vi "UV-VIS GetNumberHSSpeedsSD.vi"(4 "error in (no error)":errorcluster, 5 "type":T1, 6 "channel":i32, 7 "Control in":refnum<class "CCD_camera.lvclass">) -> (0 "error out":errorcluster, 1 "DLL error code":u32, 2 "number":i32, 3 "Control out":refnum<class "CCD_camera.lvclass">)   [LabVIEW 2020, in "CCD_camera.lvclass"]
doc: "As your AndorMCD[tm] system is capable of operating at more than one horizontal shift speed this function will return the actual number of speeds available.\n\n<B>Parameters:</B>\nchannel - the AD channel\ntype - the horizontal read mode\n Valid values: 0 - speed of data readout\n 1 - speed of binning\n 2 - speed of dumping pixels\nnumber - number of allowed horizontal speeds\n\n<B>Error codes:</B>\nDRV_SUCCESS - Speed returned.\nDRV_NOT_INITIALIZED - System not initialized.\nDRV_ACQUIRING - Acquisition in progress.\nDRV_P1INVALID - Invalid channel.\nDRV_P2INVALID - Invalid horizontal read mode."
uses:
  CCD_camera.lvclass
  atmcd32d.llb/HSSpeed_type typedef.ctl
  C:/dev/TRANCON/Classes/Detector/Detector.lvclass
  Detector.lvclass/Detector.ctl
  Detector.lvclass
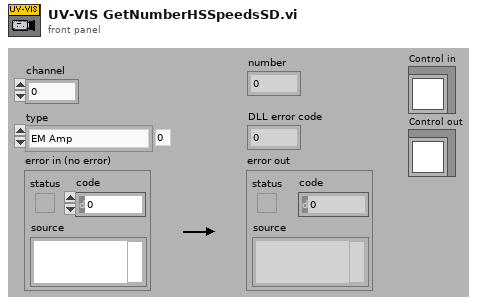
[diagram p1: front panel]
types:
  T1 = typedef "HSSpeed_type typedef.ctl" = enum16{"EM Amp", "Conventional Amp"}
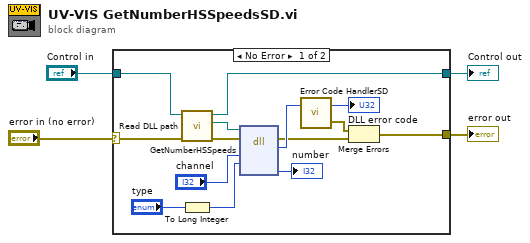
[diagram p0: block diagram]
diagram:
  n1 = case shown="No Error" "error in (no error)" {
    selector: "error in (no error)" -> [w9 w20]
    tunnel: [w6 w20] -> w3
    tunnel: [w5 w19] -> w2
    tunnel: "Control in" -> [w10 w19]
    frame No Error {
      n2 = call "Read DLL path.vi"("error in (no error)"=w9, "Detector in"=w10) -> ("error out"=w12:errorcluster, "DLL path"=w11:path, "Detector out"=w5:refnum<class "CCD_camera.lvclass">)  [unwired: 7 in]
      n3 = To Long Integer(number="type") -> (32bit integer=w14:i32)
      n4 = dll-call lib="S:/TRANCON/DLL/Atmcd32d.dll" fn="GetNumberHSSpeeds"(path in=w11, error in=w12, "channel"="channel", "type"=w14) -> (error out=w8:errorcluster, "return type"=w18:u32, "number"=→"number":i32)  [unwired: 4 in, 1 out]
      n5 = call "Error Code HandlerSD.vi"("DLL error code"=w18) -> ("error out"=w7:errorcluster, "dup DLL error code"=→"DLL error code":u32)  [unwired: 1 in]
      n6 = Merge Errors(w7, w8) -> (w6:errorcluster)
    }
    frame Error {
    }
  }
  "error out" <- w3
  "Control out" <- w2
